vi "Read Interpolate color.vi"(9 "ColorScale in":refnum<class "ColorScale.lvclass">) -> (3 "ColorScale out":refnum<class "ColorScale.lvclass">, 4 "Interpolate color":bool)   [LabVIEW 2014, in "Raspberry Pi Compatible Compiler for LabVIEW.lvlib" / "ColorScale.lvclass"]
uses:
  ColorScale.lvclass
  ColorScale.lvclass/ColorScale.ctl
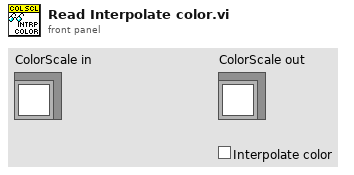
[diagram p1: front panel]
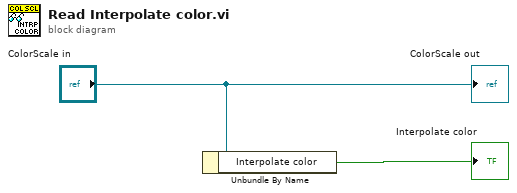
[diagram p0: block diagram]
diagram:
  n1 = Unbundle By Name("ColorScale in") -> ("Interpolate color"=→"Interpolate color":bool)
  "ColorScale out" <- "ColorScale in"
